vi "Draw Markers.vi"(7 "XYGraph in":refnum<vi>, 9 "Marker Options":T3={"Color"=16723218, "pen"={"Width"=2, "Style"=enum."Solid"}, "font"={"Font Name"="Arial", "Size"=16, "Strikeout?"=FALSE, "Italic?"=FALSE, "Underline?"=FALSE, "Outline?"=FALSE, "Shadow?"=FALSE, "Bold?"=FALSE, "FontColor"=0}, "caption"=""}, 10 "Marker":T1={"Type"=enum."vert", "X"=2.0, "Y"=2.0, "X2"=2.0, "Y2"=2.0, "Text"="Drag and click to\nposition a marker"}, 11 "picture":picture) -> (3 "new picture":picture)   [LabVIEW 2020, in "Graph Extensions.lvlib"]
doc: "Draw the appropriate line for markers, depending on the type"
uses:
  Graph Extensions.lvlib
  controls/MarkerOptions.ctl
  controls/MarkerInfo.ctl
  controls/markerType.ctl
  <vilib>/Utility/miscctls.llb/LVPoint32TypeDef.ctl
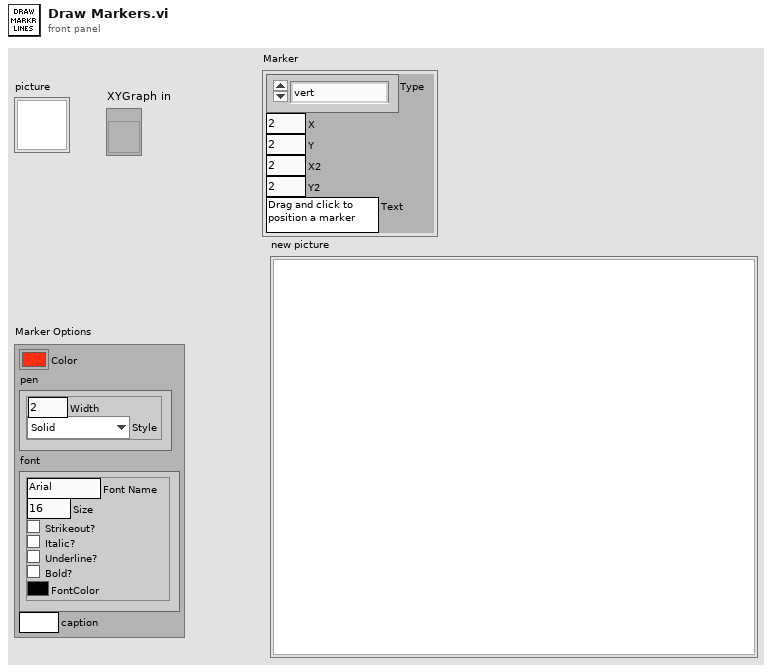
[diagram p1: front panel]
types:
  T1 = typedef "Graph Extensions.lvlib/MarkerInfo.ctl" = cluster{"Type":T2, "X":dbl, "Y":dbl, "X2":dbl, "Y2":dbl, "Text":string}
  T2 = typedef "Graph Extensions.lvlib/markerType.ctl" = enum16{"point", "arrow", "horiz", "vert", "vert range", "horiz range", "box"}
  T3 = typedef "Graph Extensions.lvlib/MarkerOptions.ctl" = cluster{"Color":u32, "pen":cluster{"Width":u16, "Style":enum32{"Solid", "Dash", "Dot", "DashDot", "DashDotDot"}}, "font":cluster{"Font Name":string, "Size":i16, "Strikeout?":bool, "Italic?":bool, "Underline?":bool, "Outline?":bool, "Shadow?":bool, "Bold?":bool, "FontColor":u32}, "caption":string}
  T4 = typedef "LVPoint32TypeDef.ctl" = cluster{"Horizontal":i32, "Vertical":i32}
  T5 = cluster{"Font Name:":string, "Size":i16, "Strikeout?":bool, "Italic?":bool, "Underline?":bool, "Outline?":bool, "Shadow?":bool, "Bold?":bool}
  T6 = enum16{"User-specified Font", "Application Font", "System Font", "Dialog Font"}
  T7 = typedef "LVRectTypeDef.ctl" = cluster{"Left":i16, "Top":i16, "Right":i16, "Bottom":i16}
  T8 = cluster{"Font Name":string, "Size":i16, "Strikeout?":bool, "Italic?":bool, "Underline?":bool, "Outline?":bool, "Shadow?":bool, "Bold?":bool, "FontColor":u32}
  T9 = cluster{"Width":u16, "Style":enum32{"Solid", "Dash", "Dot", "DashDot", "DashDotDot"}}
  T10 = cluster{"left":i16, "top":i16, "right":i16, "bottom":i16}
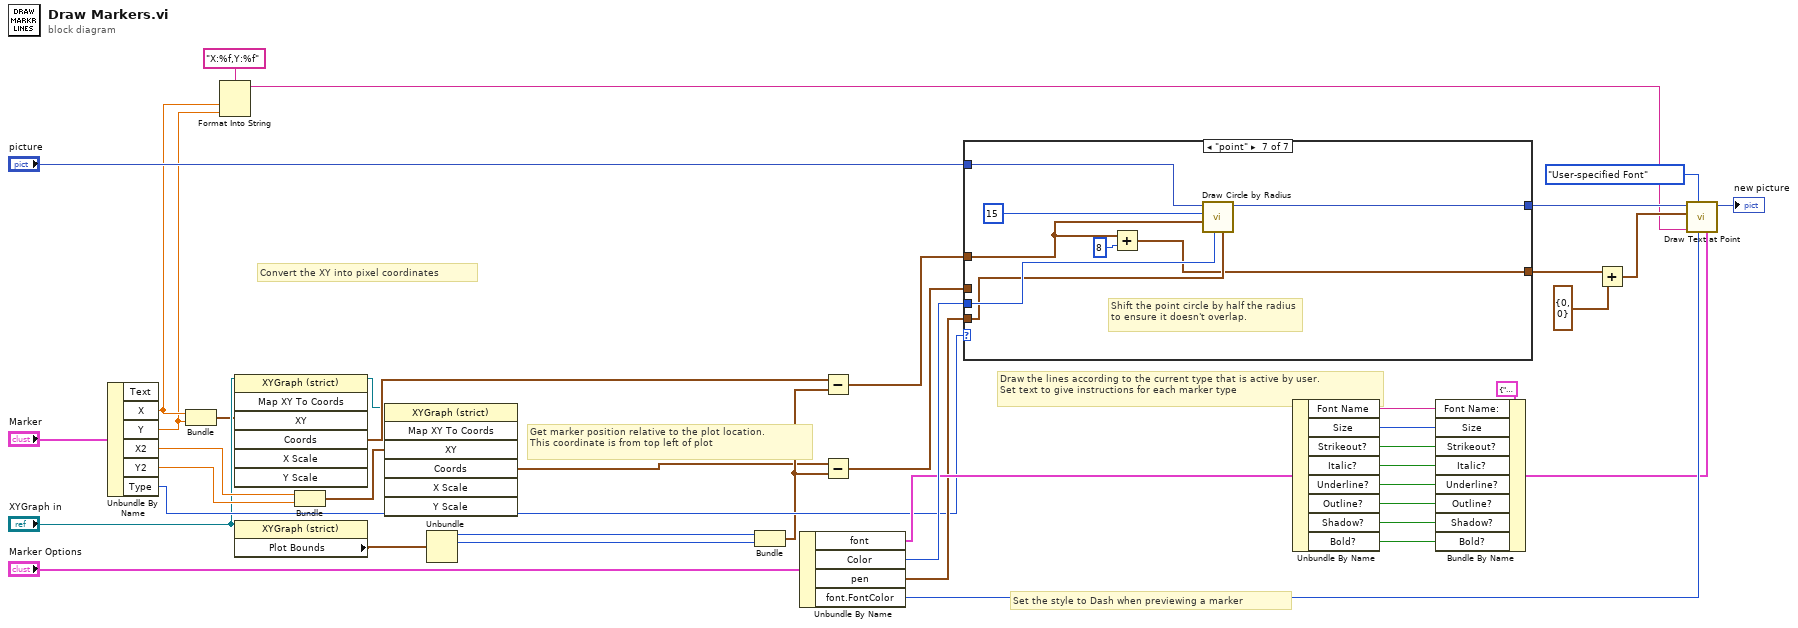
[diagram p0: block diagram]
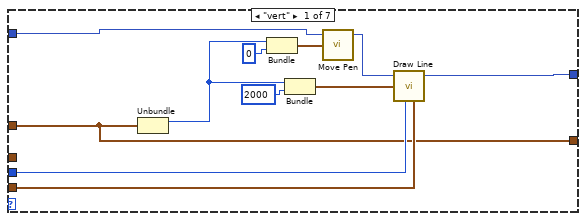
[diagram p2: hidden frame]
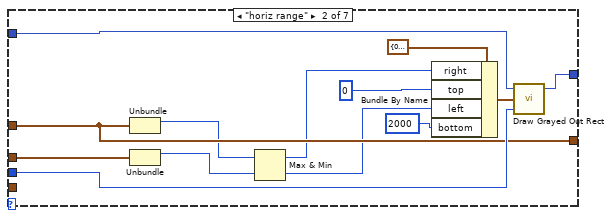
[diagram p3: hidden frame]
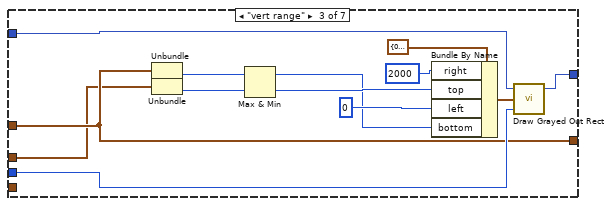
[diagram p4: hidden frame]
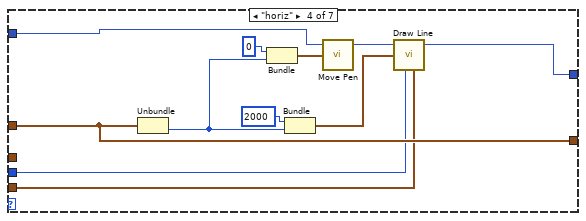
[diagram p5: hidden frame]
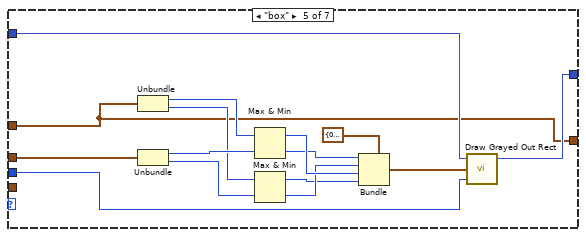
[diagram p6: hidden frame]
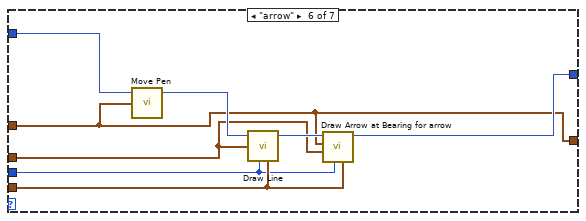
[diagram p7: hidden frame]
diagram:
  # "Convert the XY into pixel coordinates"
  # "Get marker position relative to the plot location.\nThis coordinate is from top left of plot"
  # "Set the style to Dash when previewing a marker"
  # "Draw the lines according to the current type that is active by user.\nSet text to give instructions for each marker type"
  n1 = Unbundle By Name("Marker") -> ("X"=w4:dbl, "Y"=w3:dbl, "X2"=w15:dbl, "Y2"=w14:dbl, "Type"=w16:T2)  [unwired: 1 out]
  n2 = Bundle("X"=w4, "Y"=w3) -> (w10:cluster{"X":dbl, "Y":dbl})  [unwired: 1 in]
  n3 = Format Into String(format string="X:%f,Y:%f", w4, w3) -> (resulting string=w1:string)  [unwired: 2 in, 1 out]
  n4 = invoke class="XYGraph (strict)" method="Map XY To Coords"(reference="XYGraph in", "XY"=w10) -> (reference out=w8:refnum<vi>, "Coords"=w9:T4)  [unwired: 5 in, 5 out]
  n5 = property on="Property Node" class="XYGraph (strict)"(reference="XYGraph in") -> ("Plot Bounds"=w19:T7)  [unwired: 1 in, 2 out]
  n6 = Bundle("X2"=w15, "Y2"=w14) -> (w7:cluster{"X2":dbl, "Y2":dbl})  [unwired: 1 in]
  n7 = invoke class="XYGraph (strict)" method="Map XY To Coords"(reference=w8, "XY"=w7) -> ("Coords"=w6:T4)  [unwired: 5 in, 6 out]
  n8 = Unbundle(w19) -> ("Left"=w20:i16, "Top"=w21:i16)  [unwired: 2 out]
  n9 = Bundle("Left"=w20, "Top"=w21) -> (w13:cluster{"Left":i16, "Top":i16})  [unwired: 1 in]
  n10 = Unbundle By Name("Marker Options") -> ("font"=w26:T8, "Color"=w28:u32, "pen"=w17:T9, "font.FontColor"=w39:u32)
  n11 = Subtract(x=w9, y=w13) -> (x-y=w18:T4)
  n12 = Subtract(x=w6, y=w13) -> (x-y=w12:T4)
  n13 = case shown="\"point\"" w16 {
    tunnel: w18 -> [w43 w64 w77 w83 w91 w106 w116]
    tunnel: [w51 w66 w79 w89 w103 w110 w121] -> w41
    tunnel: "picture" -> [w46 w58 w73 w80 w105 w112 w117]
    tunnel: w28 -> [w45 w65 w78 w82 w104 w108 w120]
    tunnel: w17 -> [w44 _ _ w81 _ w109 w118]
    tunnel: [w43 w64 w77 w83 w91 w106 w114] -> w27
    tunnel: w12 -> [_ w59 w74 _ w100 w107 _]
    frame "vert" {
      n14 = Unbundle(w43) -> ("Horizontal"=w53:i32)  [unwired: 1 out]
      n15 = Bundle("Horizontal"=w53, "top"=i16 0) -> (w47:cluster{"Horizontal":i32, "top":i16})  [unwired: 1 in]
      n16 = Bundle("Horizontal"=w53, "top"=i16 2000) -> (w52:cluster{"Horizontal":i32, "top":i16})  [unwired: 1 in]
      n17 = call <vilib>:"Move Pen.vi"("new position"=w47, "picture"=w46) -> ("new picture"=w50:picture)  [unwired: 3 in]
      n18 = call <vilib>:"Draw Line.vi"("picture"=w50, "end point"=w52, "color(black)"=w45, "pen"=w44) -> ("new picture"=w51:picture)  [unwired: 5 in]
    }
    frame "horiz range" {
      n19 = Unbundle(w64) -> ("Horizontal"=w57:i32)  [unwired: 1 out]
      n20 = Unbundle(w59) -> ("Horizontal"=w56:i32)  [unwired: 1 out]
      n21 = Max & Min(x=w57, y=w56) -> (max(x,y)=w54:i32, min(x,y)=w55:i32)
      n22 = Bundle By Name(cluster=T10 {"left"=0, "top"=0, "right"=0, "bottom"=0} ("rect"), "right"=w54, "top"=i16 0, "left"=w55, "bottom"=i16 2000) -> (w62:T10)
      n23 = call <vilib>:"Draw Grayed Out Rect.vi"("color(black)"=w65, "rect"=w62, "picture"=w58) -> ("new picture"=w66:picture)  [unwired: 2 in]
    }
    frame "vert range" {
      n24 = Unbundle(w77) -> ("Vertical"=w72:i32)  [unwired: 1 out]
      n25 = Unbundle(w74) -> ("Vertical"=w71:i32)  [unwired: 1 out]
      n26 = Max & Min(x=w72, y=w71) -> (max(x,y)=w67:i32, min(x,y)=w68:i32)
      n27 = Bundle By Name(cluster=T10 {"left"=0, "top"=0, "right"=0, "bottom"=0} ("rect"), "right"=i16 2000 ("top"), "top"=w68, "left"=i16 0 ("bottom"), "bottom"=w67) -> (w75:T10)
      n28 = call <vilib>:"Draw Grayed Out Rect.vi"("color(black)"=w78, "rect"=w75, "picture"=w73) -> ("new picture"=w79:picture)  [unwired: 2 in]
    }
    frame "horiz" {
      n29 = Unbundle(w83) -> ("Vertical"=w85:i32)  [unwired: 1 out]
      n30 = Bundle("top"=i16 0, "Vertical"=w85) -> (w87:cluster{"top":i16, "Vertical":i32})  [unwired: 1 in]
      n31 = Bundle("top"=i16 2000, "Vertical"=w85) -> (w90:cluster{"top":i16, "Vertical":i32})  [unwired: 1 in]
      n32 = call <vilib>:"Move Pen.vi"("new position"=w87, "picture"=w80) -> ("new picture"=w88:picture)  [unwired: 3 in]
      n33 = call <vilib>:"Draw Line.vi"("picture"=w88, "end point"=w90, "color(black)"=w82, "pen"=w81) -> ("new picture"=w89:picture)  [unwired: 5 in]
    }
    frame "box" {
      n34 = Unbundle(w91) -> ("Horizontal"=w99:i32, "Vertical"=w95:i32)
      n35 = Unbundle(w100) -> ("Horizontal"=w98:i32, "Vertical"=w94:i32)
      n36 = Max & Min(x=w99, y=w98) -> (max(x,y)=w97:i32, min(x,y)=w96:i32)
      n37 = Max & Min(x=w95, y=w94) -> (max(x,y)=w92:i32, min(x,y)=w93:i32)
      n38 = Bundle(cluster=T10 {"left"=0, "top"=0, "right"=0, "bottom"=0} ("rect"), "left"=w96, "top"=w93, "right"=w97, "bottom"=w92) -> (w102:T10)
      n39 = call <vilib>:"Draw Grayed Out Rect.vi"("color(black)"=w104, "rect"=w102, "picture"=w105) -> ("new picture"=w103:picture)  [unwired: 2 in]
    }
    frame "arrow" {
      n40 = call <vilib>:"Move Pen.vi"("new position"=w106, "picture"=w112) -> ("new picture"=w113:picture)  [unwired: 3 in]
      n41 = call <vilib>:"Draw Line.vi"("picture"=w113, "end point"=w107, "color(black)"=w108, "pen"=w109) -> ("new picture"=w111:picture)  [unwired: 5 in]
      n42 = call "Draw Arrow at Bearing for arrow.vi"("pen"=w109, "color(black)"=w108, "P2"=w107, "P1"=w106, "new picture in"=w111) -> ("new picture out"=w110:picture)  [unwired: 6 in]
    }
    frame "point" {
      # "Shift the point circle by half the radius to ensure it doesn't overlap."
      n43 = Add(x=w116, y=8 ("Horizontal")) -> (x+y=w114:T4)
      n44 = call <vilib>:"Draw Circle by Radius.vi"("pen"=w118, "color(black)"=w120, "pixel center"=w116, "radius"=i16 15, "picture"=w117) -> ("new picture"=w121:picture)  [unwired: 6 in]
    }
  }
  n45 = Unbundle By Name(w26) -> ("Font Name"=w37:string, "Size"=w36:i16, "Strikeout?"=w35:bool, "Italic?"=w34:bool, "Underline?"=w33:bool, "Outline?"=w32:bool, "Shadow?"=w31:bool, "Bold?"=w30:bool)
  n46 = Bundle By Name(cluster=T5 {"Font Name:"="", "Size"=12, "Strikeout?"=FALSE, "Italic?"=FALSE, "Underline?"=FALSE, "Outline?"=FALSE, "Shadow?"=FALSE, "Bold?"=FALSE} ("[user-specified font]"), "Font Name:"=w37, "Size"=w36, "Strikeout?"=w35, "Italic?"=w34, "Underline?"=w33, "Outline?"=w32, "Shadow?"=w31, "Bold?"=w30) -> (w29:T5)
  n47 = Add(x=w27, y=T4 {"Horizontal"=0, "Vertical"=0} ("x+y")) -> (x+y=w42:T4)
  n48 = call <vilib>:"Draw Text at Point.vi"("[user-specified font]"=w29, "text color(black)"=w39, "desired font(Application)"=T6."User-specified Font", "text"=w1, "origin"=w42, "picture"=w41) -> ("new picture"=→"new picture":picture)  [unwired: 4 in, 1 out]
